vi "Rotate.vi"(0 "reference in":refnum<class "Electric Motor.lvclass">, 5 "Degree":string, 11 "Error In":errorcluster) -> (4 "reference out":refnum<class "Electric Motor.lvclass">, 6 "Result":string, 15 "Error Out":errorcluster)   [LabVIEW 2024, in "Electric Motor.lvclass"]
uses:
  Electric Motor.lvclass
  Electric Motor.lvclass/Electric Motor.ctl
panel:
  # "Connector Pane"
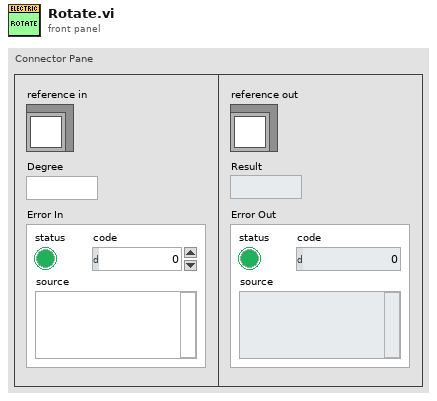
[diagram p1: front panel]
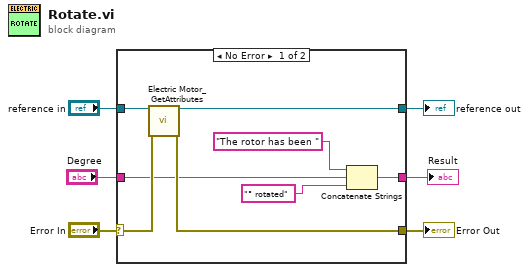
[diagram p0: block diagram]
diagram:
  n1 = case shown="No Error" "Error In" {
    selector: "Error In" -> [w14 w16]
    tunnel: [w13 w16] -> w5
    tunnel: [w11 w15] -> w3
    tunnel: "reference in" -> [w12 w15]
    tunnel: "Degree" -> [w8 _]
    tunnel: [w7 _] -> w1
    frame No Error {
      n2 = call "Electric Motor_GetAttributes.vi"("reference in"=w12, "Error In"=w14) -> ("reference out"=w11:refnum<class "Electric Motor.lvclass">, "Error Out"=w13:errorcluster)  [unwired: 10 in, 2 out]
      n3 = Concatenate Strings("The rotor has been " ("string"), w8, "° rotated" ("string")) -> (w7:string)
    }
    frame Error {
    }
  }
  "Error Out" <- w5
  "reference out" <- w3
  "Result" <- w1
